vi "Read Tag Element (String).vi"(8 "error in":errorcluster, 9 "default":string, 10 "Tag Name":string, 11 "node in":refnum<k20>) -> (0 "error out":errorcluster, 1 "value":string, 3 "node out":refnum<k20>)   [LabVIEW 2020, in "AIM ARINC 664 Import.lvlib"]
uses:
  AIM ARINC 664 Import.lvlib
  <resource>/objmgr/DOMUserDefRef.rc
  <vilib>/xml/NI_XML.lvlib
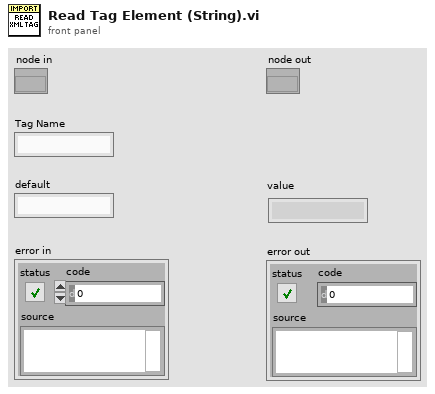
[diagram p1: front panel]
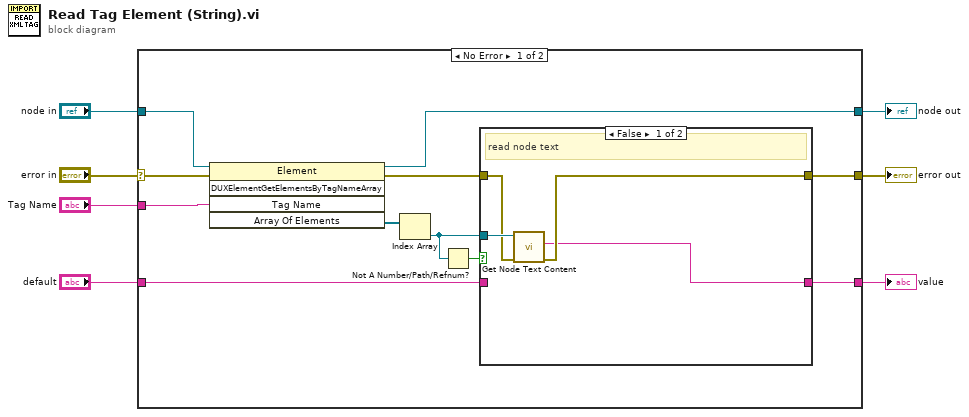
[diagram p0: block diagram]
diagram:
  n1 = case shown="No Error" "error in" {
    selector: "error in" -> [w8 w27]
    tunnel: [w18 w27] -> w7
    tunnel: "node in" -> [w14 w26]
    tunnel: "Tag Name" -> [w12 _]
    tunnel: [w11 w25] -> w4
    tunnel: [w10 w26] -> w3
    tunnel: "default" -> [w9 w25]
    frame No Error {
      n2 = invoke class="Element" method="DUXElementGetElementsByTagNameArray"(reference=w14, error in=w8, "Tag Name"=w12) -> (reference out=w10:refnum<k20>, error out=w17:errorcluster, "Array Of Elements"=w13:refnum<k20>[])  [unwired: 2 in, 2 out]
      n3 = Index Array(array=w13) -> (element=w15:refnum<k20>)  [unwired: 1 in]
      n4 = Not A Number/Path/Refnum?(number/path/refnum=w15) -> (NaN/Path/Refnum?=w16:bool)
      n5 = case shown="False" w16 {
        tunnel: w15 -> [w22 _]
        tunnel: w17 -> [w21 w24]
        tunnel: [w19 w23] -> w11
        tunnel: [w20 w24] -> w18
        tunnel: w9 -> [_ w23]
        frame False {
          # "read node text"
          n6 = call <vilib>:"Get Node Text Content.vi"("error in (no error)"=w21, "node in"=w22) -> ("error out"=w20:errorcluster, "node text"=w19:string)  [unwired: 7 in, 1 out]
        }
        frame True {
          # "pass default if element doesn't exist"
        }
      }
    }
    frame Error {
    }
  }
  "error out" <- w7
  "node out" <- w3
  "value" <- w4
